vi "getActionPanelPath.vi"(8 "error in (no error)":errorcluster, 11 "rfAction in":refnum<class "rfAction.lvclass">) -> (0 "error out":errorcluster, 2 "frontPanelPath":path, 3 "rfAction out":refnum<class "rfAction.lvclass">)   [LabVIEW 2011, in "Views.lvlib" / "ScriptEditor.lvlib" / "rfAction.lvclass"]
uses:
  rfAction.lvclass
  Tools/Filing/FileSystem/FileSystem.lvclass
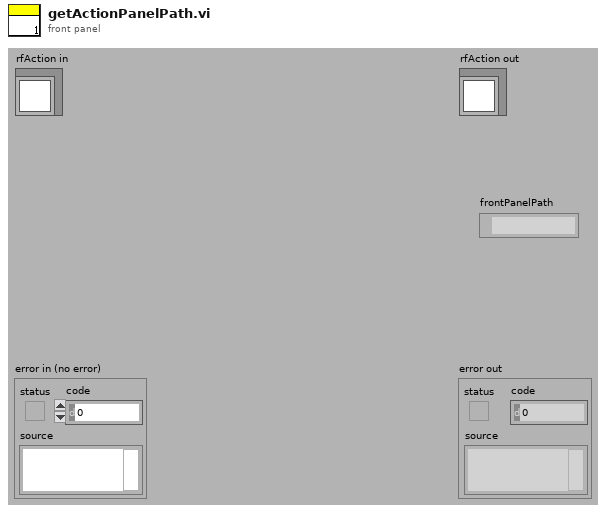
[diagram p1: front panel]
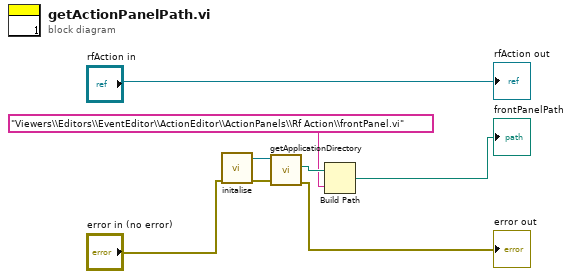
[diagram p0: block diagram]
diagram:
  n1 = call "initalise.vi"("error in (no error)"="error in (no error)") -> ("error out"=w8:errorcluster, "FileSystem out"=w7:refnum<class "FileSystem.lvclass">)  [unwired: 9 in]
  n2 = call-dynamic "getApplicationDirectory.vi"("error in (no error)"=w8, "FileSystem.lvclass in"=w7) -> ("error out"=→"error out":errorcluster, "ApplicationDirectory"=w6:path)  [unwired: 7 in, 1 out]
  n3 = Build Path(base path=w6, name or relative path="Viewers\\Editors\\EventEditor\\ActionEditor\\ActionPanels\\Rf Action\\frontPanel.vi") -> (appended path=→"frontPanelPath":path)
  "rfAction out" <- "rfAction in"
